vi "frecuency-pwm-calculator.vi"() -> ()   [LabVIEW 2013]
uses:
  <vilib>/Waveform/DWDTOps.llb/DWDT Boolean Array to Digital.vi
panel:
  in  "Puntos por ciclo (resolucion)":dbl=100.0 format="%#_13g"
  out "PWM digital shape":digitalwaveform(waveform)={"t0"=timestamp(0 s since 1904-01-01), "dt"=0.0, "Y"={"transitions"=[], "data"=[]}, "error"={"status"=FALSE, "code"=37421928, "source"=""}}
  out "Frecuencia de la base de tiempos":dbl
  out "Duty cycle increment values":dbl
  in  "Periodo de muestreo":dbl=0.2
  in  "Numero de pulsos por muestreo (N)":dbl=4.0
  in  "Duty Cycle":dbl=1.0 min=0.0 max=100.0 step=0.01 format="%#_5g"
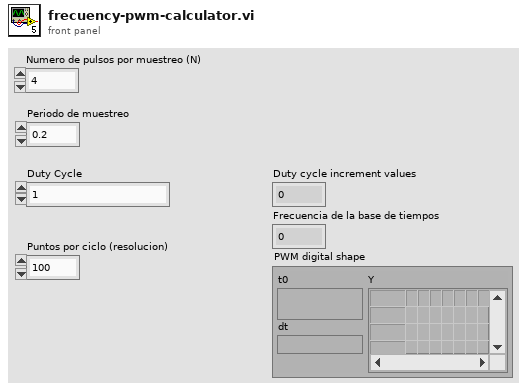
[diagram p1: front panel]
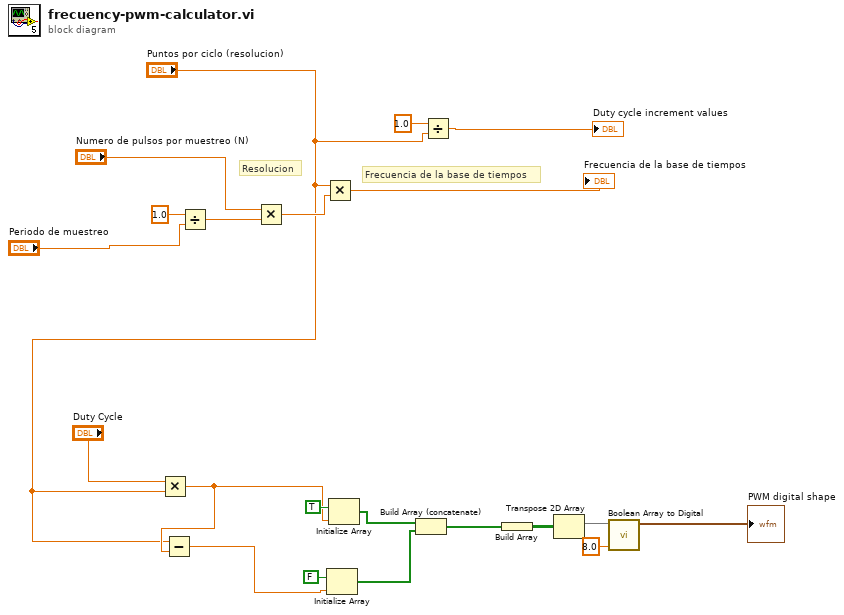
[diagram p0: block diagram]
diagram:
  # "Resolucion"
  # "Frecuencia de la base de tiempos"
  n1 = Multiply(x="Duty Cycle", y="Puntos por ciclo (resolucion)") -> (x*y=w10:dbl)
  n2 = Subtract(x="Puntos por ciclo (resolucion)", y=w10) -> (x-y=w9:dbl)
  n3 = Divide(x=1.0, y="Periodo de muestreo") -> (x/y=w20:dbl)
  n4 = Multiply(x="Numero de pulsos por muestreo (N)", y=w20) -> (x*y=w19:dbl)
  n5 = Multiply(x="Puntos por ciclo (resolucion)", y=w19) -> (x*y=→"Frecuencia de la base de tiempos":dbl)
  n6 = Initialize Array(FALSE, w9) -> (w12:bool[])
  n7 = Initialize Array(TRUE, w10) -> (w14:bool[])
  n8 = Build Array (concatenate)(w14, w12) -> (w7:bool[])
  n9 = Divide(x=1.0, y="Puntos por ciclo (resolucion)") -> (x/y=→"Duty cycle increment values":dbl)
  n10 = Build Array(w7) -> (w6:bool[][])
  n11 = Transpose 2D Array(2D array=w6) -> (transposed array=w8:bool[][])
  n12 = call-poly <vilib>:"Boolean Array to Digital.vi"("sample rate"=8.0, "boolean array"=w8) -> ("digital waveform"=→"PWM digital shape":digitalwaveform)  [unwired: 8 in, 1 out]
